vi "get_position.vi"(8 "error in (no error)":errorcluster, 11 "Newport Model 8742 in":refnum<class "Newport Model 8742.lvclass">) -> (0 "error out":errorcluster, 2 "Position (steps)":i32, 3 "Newport Model 8742 out":refnum<class "Newport Model 8742.lvclass">)   [LabVIEW 2020, in "Newport Model 8742.lvclass"]
uses:
  Newport Model 8742.lvclass
  Newport Model 8742.lvclass/Newport Model 8742.ctl
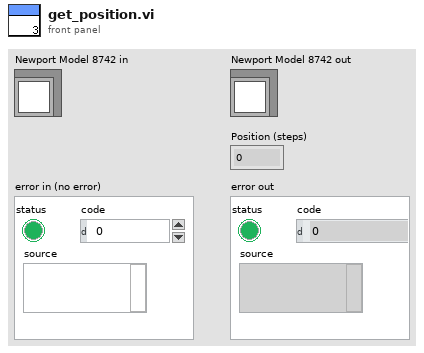
[diagram p1: front panel]
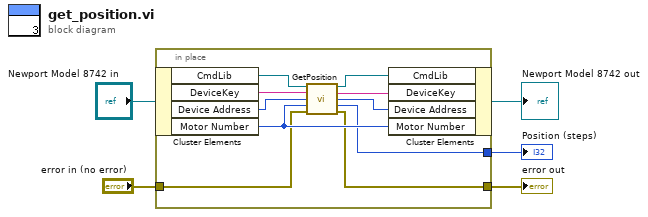
[diagram p0: block diagram]
diagram:
  n1 = in-place {
    in-place-border: "error in (no error)" -> [w11]
    in-place-border: [w10] -> w2
    in-place-border: [w7] -> w3
    n2 = in-place-cluster #1("Newport Model 8742 in") -> ("CmdLib"=w15:refnum<k24>, "DeviceKey"=w14:string, "Device Address"=w13:i32, "Motor Number"=w12:i32)
    n3 = call <instrlib>:"GetPosition.vi"("CmdLib In"=w15, "DeviceKey In"=w14, "Device Address In"=w13, "Motor"=w12, "error in (no error)"=w11) -> ("CmdLib Out"=w8:refnum<k24>, "DeviceKey Out"=w9:string, "Device Address Out"=w6:i32, "Position"=w7:i32, "error out"=w10:errorcluster)  [unwired: 6 in]
    n4 = in-place-cluster #1("CmdLib"=w8, "DeviceKey"=w9, "Device Address"=w6, "Motor Number"=w12) -> (→"Newport Model 8742 out":refnum<class "Newport Model 8742.lvclass">)
  }
  "error out" <- w2
  "Position (steps)" <- w3
